vi "test - Get Filter Configuration String - 1.vi"(8 "error in (no error)":errorcluster, 11 "TestCase in":refnum<class "String Filter Tester.lvclass">) -> (0 "error out":errorcluster, 3 "TestCase out":refnum<class "String Filter Tester.lvclass">)   [LabVIEW 2016, in "String Filter Tester.lvclass"]
uses:
  String Filter Tester.lvclass
  Core/Assert API Components/Filter Configurations/String Filters/String Filters.lvclass
  C:/Users/ukhornp/Documents/Work/Projects/actor_assert_api/Core/Assert API Components/Filter Configurations/Base Filter.lvclass
  Core/Assert API Components/Filter Configurations/Base Filter.lvclass/Base Filter.ctl
  <vilib>/addons/_JKI Toolkits/VI Tester/TestCase.llb/TestCase.lvclass
  Core/Assert API Components/Filter Configurations/Base Filter.lvclass
  C:/Program Files (x86)/National Instruments/LabVIEW 2016/vi.lib/addons/_JKI Toolkits/VI Tester/TestCase.llb/TestCase.lvclass
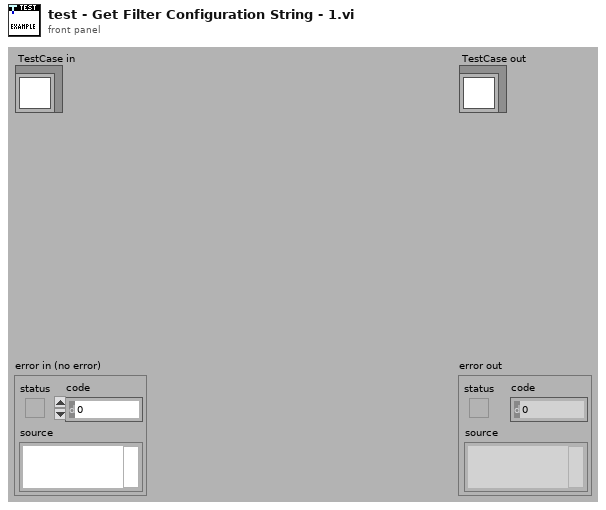
[diagram p1: front panel]
types:
  T1 = enum16{"Contains", "Does Not Contain", "Starts With", "Equals", "Does Not Equal"}
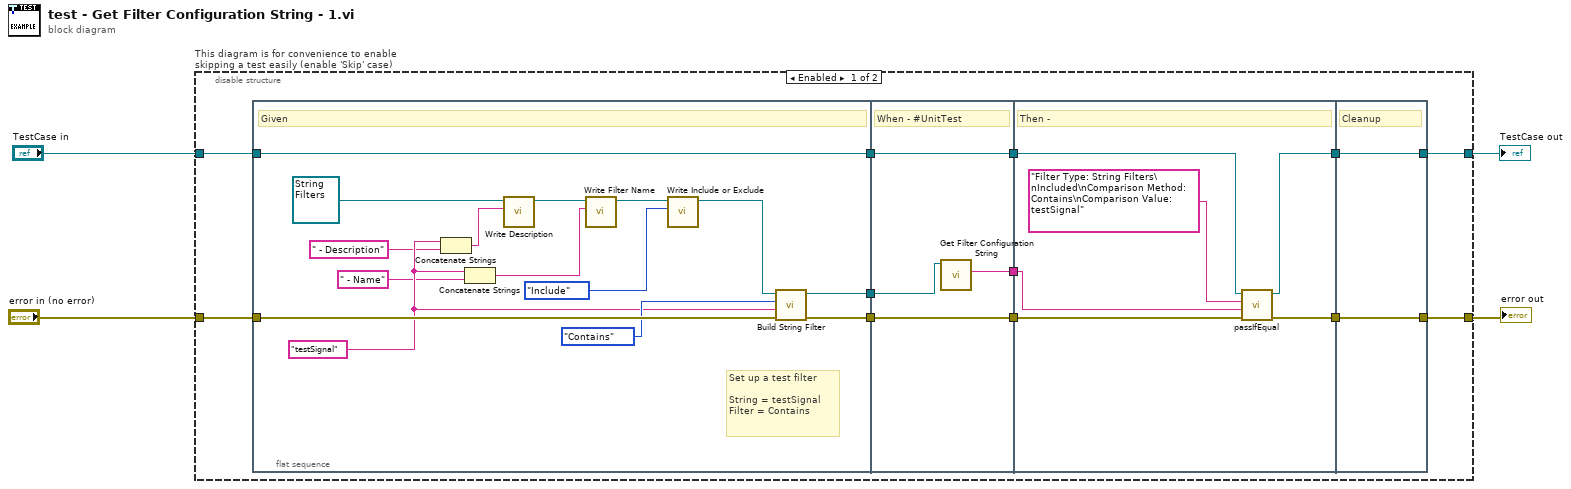
[diagram p0: block diagram]
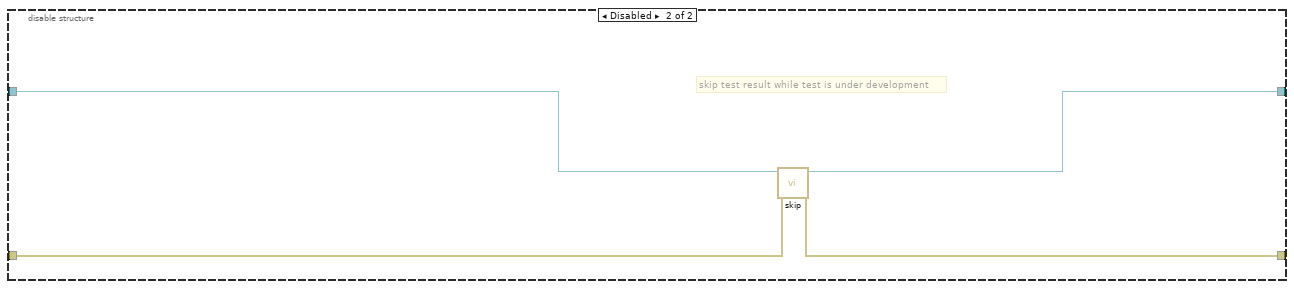
[diagram p2: hidden frame]
diagram:
  n1 = disable-structure "This diagram is for convenience to enable skipping a test easily (enable 'Skip' case)" shown="Enabled" {
    disable-tunnel: "TestCase in" -> [w10 w47]
    disable-tunnel: [w7 w45] -> w1
    disable-tunnel: [w8 w46] -> w3
    disable-tunnel: "error in (no error)" -> [w9 w44]
    frame Enabled {
      n2 = flat-sequence {
        tunnel: w9 -> [w30]
        tunnel: w10 -> [w31]
        tunnel: [w31] -> w16
        tunnel: [w29] -> w15
        tunnel: [w26] -> w6
        tunnel: [w35] -> w14
        tunnel: [w34] -> w13
        tunnel: w16 -> [w35]
        tunnel: w15 -> [w34]
        tunnel: w6 -> [w33]
        tunnel: [w32] -> w5
        tunnel: [w40] -> w12
        tunnel: [w38] -> w11
        tunnel: w14 -> [w41]
        tunnel: w13 -> [w39]
        tunnel: w5 -> [w36]
        tunnel: [w42] -> w8
        tunnel: [w43] -> w7
        tunnel: w12 -> [w43]
        tunnel: w11 -> [w42]
        frame #0 {
          w22 = "testSignal" ("Comparison Value")
          # "Set up a test filter\n\nString = testSignal \nFilter = Contains"
          # "Given"
          n3 = Concatenate Strings(w22, " - Description" ("string")) -> (w19:string)
          n4 = Concatenate Strings(w22, " - Name" ("string")) -> (w18:string)
          n5 = call "Write Description.vi"("Description"=w19, "Base Filter in"=refnum<class "String Filters.lvclass"> refnum ("String Filters in")) -> ("Base Filter out"=w25:refnum<class "String Filters.lvclass">)  [unwired: 9 in]
          n6 = call "Write Filter Name.vi"("Filter Name"=w18, "Base Filter in"=w25) -> ("Base Filter out"=w24:refnum<class "String Filters.lvclass">)  [unwired: 9 in]
          n7 = call "Write Include or Exclude.vi"("Include or Exclude"=enum16{"Include", "Exclude"}."Include", "Base Filter in"=w24) -> ("Base Filter out"=w23:refnum<class "String Filters.lvclass">)  [unwired: 9 in]
          n8 = call-dynamic "Build String Filter.vi"("error in (no error)"=w30, "Comparison Value"=w22, "Comparison Method"=T1."Contains", "String Filters in"=w23) -> ("error out"=w29:errorcluster, "String Filters out"=w26:refnum<class "String Filters.lvclass">)  [unwired: 6 in]
        }
        frame #1 {
          # "When - #UnitTest"
          n9 = call "Get Filter Configuration String.vi"("Base Filter in"=w33) -> ("Filter Configuration"=w32:string)  [unwired: 10 in]
        }
        frame #2 {
          # "Then -"
          n10 = call-dynamic "passIfEqual.vi"("error in (no error)"=w39, "y"=w36, "x"="Filter Type: String Filters\nIncluded\nComparison Method: Contains\nComparison Value: testSignal" ("Filter Configuration"), "TestCase in"=w41) -> ("error out"=w38:errorcluster, "TestCase out"=w40:refnum<class "String Filter Tester.lvclass">)  [unwired: 6 in]
        }
        frame #3 {
          # "Cleanup"
        }
      }
    }
    frame Disabled {
      # "skip test result while test is under development"
      n11 = call <vilib>:"skip.vi"("error in (no error)"=w44, "TestCase in"=w47) -> ("error out"=w46:errorcluster, "TestCase out"=w45:refnum<class "String Filter Tester.lvclass">)  [unwired: 8 in]
    }
  }
  "error out" <- w3
  "TestCase out" <- w1
